vi "设置窗口.vi"(8 "error in (no error)":errorcluster, 11 "Cleaningcycle in":refnum<class "Cleaning cycle.lvclass">) -> (0 "error out":errorcluster, 3 "Cleaningcycle out":refnum<class "Cleaning cycle.lvclass">)   [LabVIEW 2022 SP3, in "Cleaning cycle.lvclass"]
uses:
  Cleaning cycle.lvclass
  Cleaning cycle.lvclass/Cleaning cycle.ctl
panel:
  in  "保存按钮":bool
  in  "清空按钮":bool
  in  "删除按钮":bool
  in  "添加按钮":bool
  in  "任务列表":i32[](listbox)
  in  "启用":bool
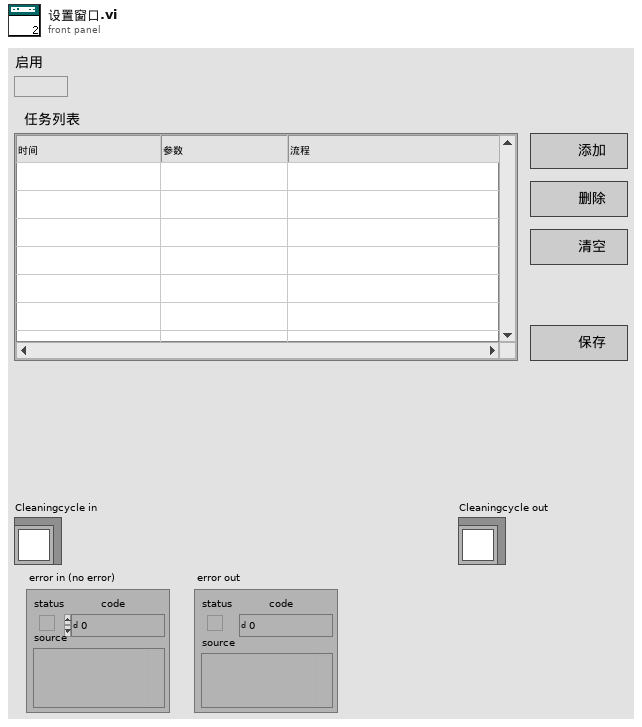
[diagram p1: front panel]
types:
  T1 = typedef "Cleaning cycle.lvclass/State Data.ctl" = cluster{"配置文件路径":path, "简易流程路径":path, "参数列表":cluster{"String":string, "Value":u16}[], "简易流程列表":cluster{"String":string, "Value":u16}[], "配置信息":T2, "命令":cluster{"触发":bool, "周期项":T4}[]}
  T2 = typedef "Cleaning cycle.lvclass/配置信息.ctl" = cluster{"任务列表":T3}
  T3 = typedef "Cleaning cycle.lvclass/任务.ctl" = cluster{"启用":bool, "项":string[][]}
  T4 = typedef "Cleaning cycle.lvclass/周期项.ctl" = cluster{"时":i32, "分":i32, "频次":string, "id":i32, "参数":string, "simpleflowid":i32, "简易流程名称":string}
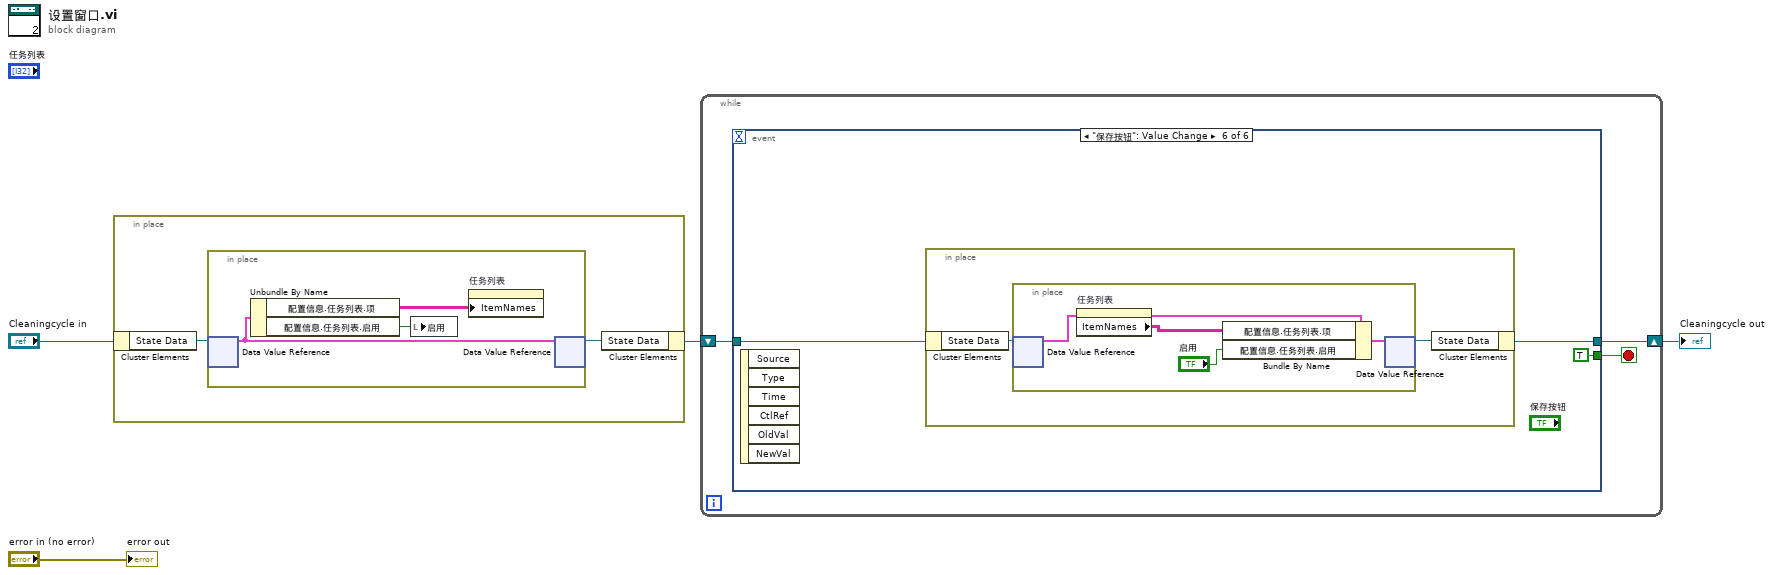
[diagram p0: block diagram]
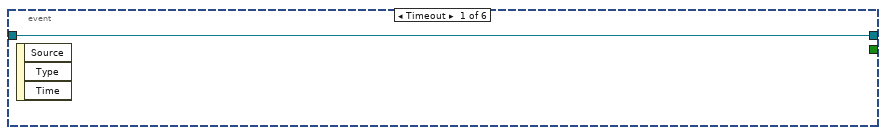
[diagram p2: hidden frame]
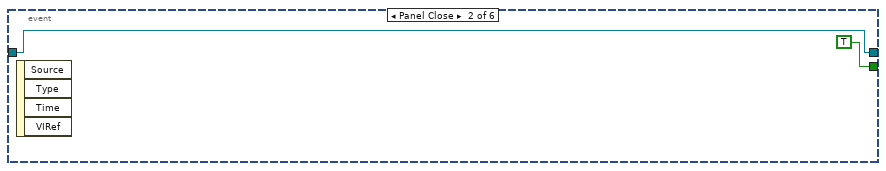
[diagram p3: hidden frame]
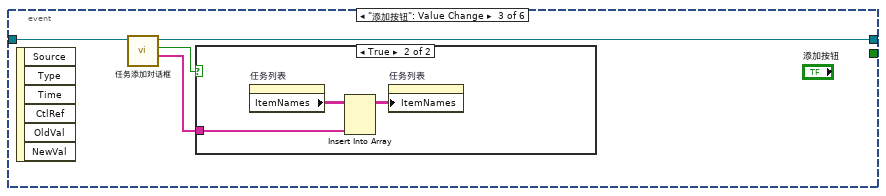
[diagram p4: hidden frame]
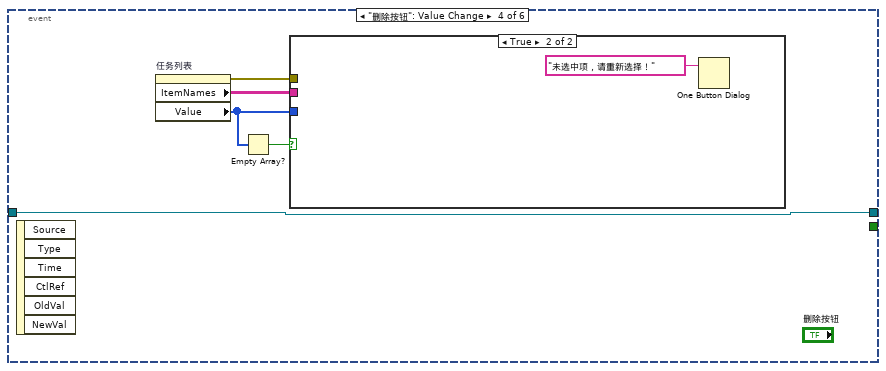
[diagram p6: hidden frame]
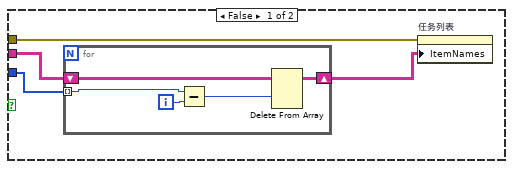
[diagram p7: hidden frame]
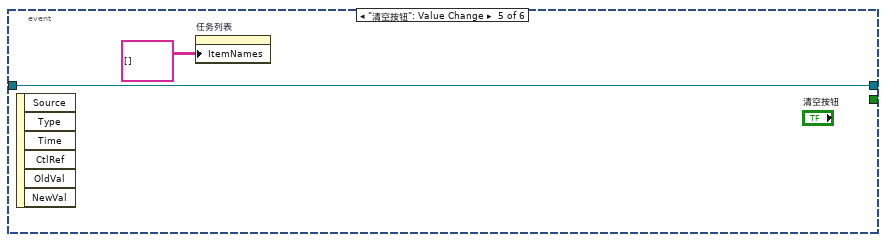
[diagram p8: hidden frame]
diagram:
  n1 = in-place {
    n2 = in-place-cluster #1("Cleaningcycle in") -> ("State Data"=w6:refnum<data-value>)
    n3 = in-place {
      n4 = in-place-dvr #2(w6) -> (w8:T1)  [unwired: 1 out]
      n5 = Unbundle By Name(w8) -> ("配置信息.任务列表.项"=w7:string[][], "配置信息.任务列表.启用"=w9:bool)
      n6 = local write "启用"(w9) -> ()
      n7 = property on="任务列表" class="MCListbox (strict)"("ItemNames"=w7) -> ()  [unwired: 2 in, 2 out]
      n8 = in-place-dvr #2(w8) -> (w5:refnum<data-value>)  [unwired: 1 out]
    }
    n9 = in-place-cluster #1("State Data"=w5) -> (w3:refnum<class "Cleaning cycle.lvclass">)
  }
  n10 = while {
    shift-right: [w10] -> w2
    shift-left: w3 -> [w11]
    stop <- w12 stop-if-true
    n11 = event shown="[5] \"保存按钮\": Value Change" {
      selector: _ -> [_ _ _ _ _ _]
      dyn-events: _ -> [_ _ _ _ _ _]
      timeout: _ -> [_ _ _ _ _ _]
      tunnel: [_ TRUE _ _ _ TRUE] -> w12
      tunnel: w11 -> [w13 w14 w19 w23 w38 w42]
      tunnel: [w13 w14 w17 w23 w38 w41] -> w10
      event Timeout {
        n12 = event-data() -> ()  [unwired: 1 in, 3 out]
      }
      event Panel Close {
        n13 = event-data() -> ()  [unwired: 1 in, 4 out]
      }
      event "添加按钮": Value Change {
        n14 = event-data() -> ()  [unwired: 1 in, 6 out]
        n15 = call "任务添加对话框.vi"("Cleaningcycle in"=w19) -> ("项名"=w16:string[], "check?"=w18:bool, "Cleaningcycle out"=w17:refnum<class "Cleaning cycle.lvclass">)  [unwired: 7 in, 1 out]
        n16 = case shown="True" w18 {
          tunnel: w16 -> [_ w20]
          frame False {
          }
          frame True {
            n17 = property on="任务列表" class="MCListbox (strict)"() -> ("ItemNames"=w22:string[][])  [unwired: 2 in, 2 out]
            n18 = Insert Into Array(array=w22, new element=w20) -> (w21:string[][])  [unwired: 2 in]
            n19 = property on="任务列表" class="MCListbox (strict)"("ItemNames"=w21) -> ()  [unwired: 2 in, 2 out]
          }
        }
      }
      event "删除按钮": Value Change {
        n20 = event-data() -> ()  [unwired: 1 in, 6 out]
        n21 = property on="任务列表" class="MCListbox (strict)"() -> (error out=w26:errorcluster, "ItemNames"=w27:string[][], "Value"=w24:i32[])  [unwired: 2 in, 1 out]
        n22 = Empty Array?(array=w24) -> (empty?=w25:bool)
        n23 = case shown="True" w25 {
          tunnel: w27 -> [w31 _]
          tunnel: w26 -> [w30 _]
          tunnel: w24 -> [w28 _]
          frame False {
            n24 = for {
              shift-right: [w35] -> w29
              shift-left: w31 -> [w36]
              tunnel: w28 -> [w34] mode=indexing
              i -> [w33]
              n25 = Subtract(x=w34, y=w33) -> (x-y=w32:i32)
              n26 = Delete From Array(array=w36, index (row)=w32) -> (array with subset deleted=w35:string[][])  [unwired: 2 in, 1 out]
            }
            n27 = property on="任务列表" class="MCListbox (strict)"(error in=w30, "ItemNames"=w29) -> ()  [unwired: 1 in, 2 out]
          }
          frame True {
            n28 = One Button Dialog(message="未选中项，请重新选择！" ("消息")) -> ()  [unwired: 1 in, 1 out]
          }
        }
      }
      event "清空按钮": Value Change {
        n29 = event-data() -> ()  [unwired: 1 in, 6 out]
        n30 = property on="任务列表" class="MCListbox (strict)"("ItemNames"=string[][] [] ("项名")) -> ()  [unwired: 2 in, 2 out]
      }
      event "保存按钮": Value Change {
        n31 = event-data() -> ()  [unwired: 1 in, 6 out]
        n32 = in-place {
          n33 = in-place-cluster #3(w42) -> ("State Data"=w44:refnum<data-value>)
          n34 = in-place {
            n35 = in-place-dvr #4(w44) -> (w48:T1)  [unwired: 1 out]
            n36 = property on="任务列表" class="MCListbox (strict)"() -> ("ItemNames"=w45:string[][])  [unwired: 2 in, 2 out]
            n37 = Bundle By Name(cluster=w48, "配置信息.任务列表.项"=w45, "配置信息.任务列表.启用"="启用") -> (w47:T1)
            n38 = in-place-dvr #4(w47) -> (w43:refnum<data-value>)  [unwired: 1 out]
          }
          n39 = in-place-cluster #3("State Data"=w43) -> (w41:refnum<class "Cleaning cycle.lvclass">)
        }
      }
    }
  }
  "Cleaningcycle out" <- w2
  "error out" <- "error in (no error)"
